vi "PostBuild.vi"(5 "Files Generated\nby Build":path[](array[path]), 6 "Top Level/Always Included VIs":path[](array[path]), 7 "Destination Path":path, 8 "error in (no error)":errorcluster, 9 "Target Name":string, 10 "Build Specification\nName":string, 11 "Project Path":path) -> (0 "error out":errorcluster)   [LabVIEW 2018]
uses:
  References/SFTP Library/Connection Info..cluster.ctl
  References/SFTP Library/LabSFTP.lvlib
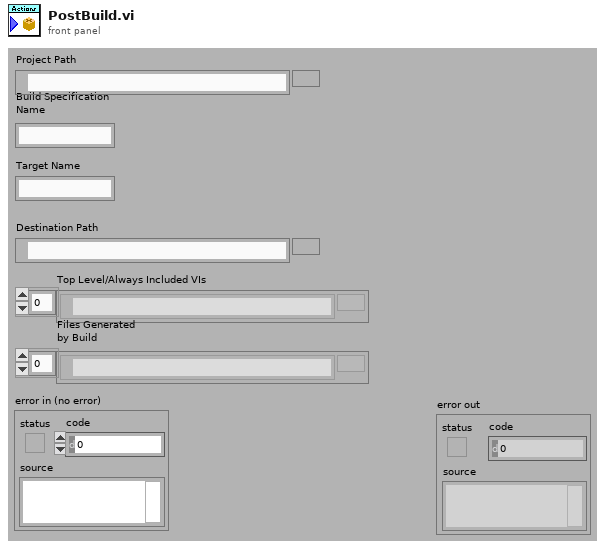
[diagram p1: front panel]
types:
  T1 = cluster{"FPGA Spec Name":string, "private key rel path":string, "Build Spec Name":string, "Project Path":path, "Destination Path":path}
  T2 = typedef "LabSFTP.lvlib/Connection Info..cluster.ctl" = cluster{"Remote":string, "Username":string, "Port (22)":i32}
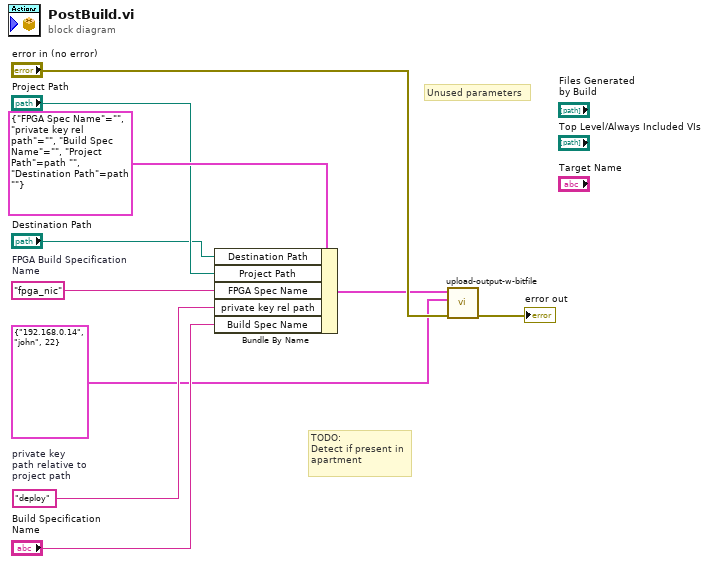
[diagram p0: block diagram]
diagram:
  w7 = "fpga_nic"  # FPGA Build Specification Name
  w6 = "deploy"  # private key path relative to project path
  # "TODO:\nDetect if present in\napartment"
  # "Unused parameters"
  n1 = Bundle By Name(cluster=T1 {"FPGA Spec Name"="", "private key rel path"="", "Build Spec Name"="", "Project Path"=path "", "Destination Path"=path ""} ("input cluster"), "Destination Path"="Destination Path", "Project Path"="Project Path", "FPGA Spec Name"=w7, "private key rel path"=w6, "Build Spec Name"="Build Specification\nName") -> (w2:T1)
  n2 = call "upload-output-w-bitfile.vi"("error in (no error)"="error in (no error)", "Connection Info."=T2 {"Remote"="192.168.0.14", "Username"="john", "Port (22)"=22}, "input cluster"=w2) -> ("error out"=→"error out":errorcluster)  [unwired: 8 in]
